vi "EncoderGetValues.vi"() -> ()   [LabVIEW 2014]
uses:
  <vilib>/Analysis/baseanly.llb/Mean (DBL).vi
  encoderData.vi
  <vilib>/Analysis/NI_AALBase.lvlib
panel:
  out "Waveform Chart":dbl(graph)
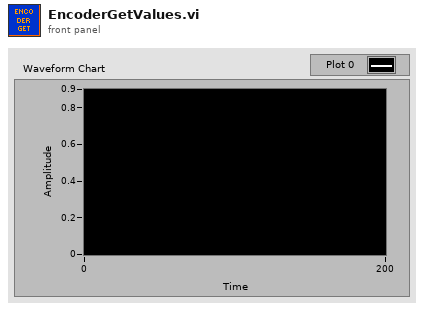
[diagram p1: front panel]
types:
  T1 = typedef "WPI_EncoderDevRef.ctl" = cluster{"DevStatus":errorcluster, "EncoderIndex":T2, "CounterIndex":T3, "DistancePerCount":dbl, "Decoding Type":T4}
  T2 = typedef "FPGA_EncoderIdx.ctl" = enum8{"Enc 0", "Enc 1", "Enc 2", "Enc 3", "Enc 4", "Enc 5", "Enc 6", "Enc 7", "Invalid"}
  T3 = typedef "FPGA_CounterCtrSystemIndex.ctl" = enum8{"Ctr 0", "Ctr 1", "Ctr 2", "Ctr 3", "Ctr 4", "Ctr 5", "Ctr 6", "Ctr 7", "Invalid"}
  T4 = typedef "WPI_EncoderType.ctl" = enum16{"1x", "2x", "4x"}
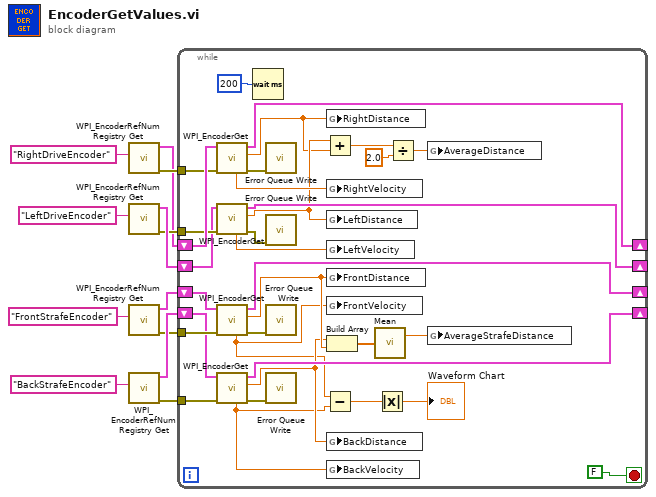
[diagram p0: block diagram]
diagram:
  n1 = call <vilib>:"WPI_EncoderRefNum Registry Get.vi"("refnum name"="RightDriveEncoder") -> ("error out"=w11:errorcluster, "EncoderDevRef"=w4:T1)  [unwired: 9 in]
  n2 = call <vilib>:"WPI_EncoderRefNum Registry Get.vi"("refnum name"="LeftDriveEncoder") -> ("error out"=w5:errorcluster, "EncoderDevRef"=w12:T1)  [unwired: 9 in]
  n3 = call <vilib>:"WPI_EncoderRefNum Registry Get.vi"("refnum name"="FrontStrafeEncoder") -> ("error out"=w8:errorcluster, "EncoderDevRef"=w7:T1)  [unwired: 9 in]
  n4 = call <vilib>:"WPI_EncoderRefNum Registry Get.vi"("refnum name"="BackStrafeEncoder") -> ("error out"=w10:errorcluster, "EncoderDevRef"=w9:T1)  [unwired: 9 in]
  n5 = while {
    shift-right: [w44] -> _
    shift-left: w4 -> [w45]
    tunnel: w5 -> [w42]
    tunnel: w8 -> [w39]
    tunnel: w10 -> [w37]
    tunnel: w11 -> [w34]
    shift-right: [w32] -> _
    shift-left: w12 -> [w33]
    shift-right: [w26] -> _
    shift-left: w7 -> [w40]
    shift-right: [w31] -> _
    shift-left: w9 -> [w38]
    stop <- FALSE stop-if-true
    n6 = call <vilib>:"WPI_EncoderGet.vi"("error in (no error)"=w34, "EncoderDevRef"=w45) -> ("error out"=w30:errorcluster, "Distance"=w24:dbl, "EncoderDevRef"=w44:T1, "Rate"=w43:dbl)  [unwired: 4 in, 2 out]
    n7 = call <vilib>:"WPI_EncoderGet.vi"("error in (no error)"=w42, "EncoderDevRef"=w33) -> ("error out"=w29:errorcluster, "Distance"=w25:dbl, "EncoderDevRef"=w32:T1, "Rate"=w41:dbl)  [unwired: 4 in, 2 out]
    n8 = call <vilib>:"WPI_EncoderGet.vi"("error in (no error)"=w39, "EncoderDevRef"=w40) -> ("error out"=w28:errorcluster, "Distance"=w18:dbl, "EncoderDevRef"=w26:T1, "Rate"=w16:dbl)  [unwired: 4 in, 2 out]
    n9 = call <vilib>:"WPI_EncoderGet.vi"("error in (no error)"=w37, "EncoderDevRef"=w38) -> ("error out"=w27:errorcluster, "Distance"=w17:dbl, "EncoderDevRef"=w31:T1, "Rate"=w15:dbl)  [unwired: 4 in, 2 out]
    n10 = Wait (ms)(milliseconds to wait=u32 200) -> ()  [unwired: 1 out]
    n11 = call "Error Queue Write.vi"("error in (no error)"=w30) -> ()  [unwired: 11 in]
    n12 = call "Error Queue Write.vi"("error in (no error)"=w29) -> ()  [unwired: 11 in]
    n13 = call "Error Queue Write.vi"("error in (no error)"=w28) -> ()  [unwired: 11 in]
    n14 = call "Error Queue Write.vi"("error in (no error)"=w27) -> ()  [unwired: 11 in]
    n15 = Add(x=w25, y=w24) -> (x+y=w23:dbl)
    n16 = Subtract(x=w16, y=w15) -> (x-y=w14:dbl)
    n17 = global write "encoderData.vi" "RightDistance"(w24) -> ()
    n18 = global write "encoderData.vi" "RightVelocity"(w43) -> ()
    n19 = global write "encoderData.vi" "LeftDistance"(w25) -> ()
    n20 = global write "encoderData.vi" "LeftVelocity"(w41) -> ()
    n21 = global write "encoderData.vi" "FrontDistance"(w18) -> ()
    n22 = global write "encoderData.vi" "FrontVelocity"(w16) -> ()
    n23 = Build Array(w17, w18) -> (w21:dbl[])
    n24 = global write "encoderData.vi" "BackDistance"(w17) -> ()
    n25 = global write "encoderData.vi" "BackVelocity"(w15) -> ()
    n26 = call-poly <vilib>:"Mean.vi"("X"=w21) -> ("mean"=w19:dbl)  [unwired: 1 out]
    n27 = Absolute Value(x=w14) -> (abs(x)=→"Waveform Chart":dbl)
    n28 = Divide(x=w23, y=2.0) -> (x/y=w20:dbl)
    n29 = global write "encoderData.vi" "AverageDistance"(w20) -> ()
    n30 = global write "encoderData.vi" "AverageStrafeDistance"(w19) -> ()
  }
